vi "setRampTime.vi"(8 "error in (no error)":errorcluster, 10 "rampTime":dbl, 11 "RfRamp in":refnum<class "RfRamp.lvclass">) -> (0 "error out":errorcluster, 3 "RfRamp out":refnum<class "RfRamp.lvclass">)   [LabVIEW 2011, in "Tools.lvlib" / "Scripting.lvlib" / "RfRamp.lvclass"]
uses:
  RfRamp.lvclass
  RfRamp.lvclass/RfRamp.ctl
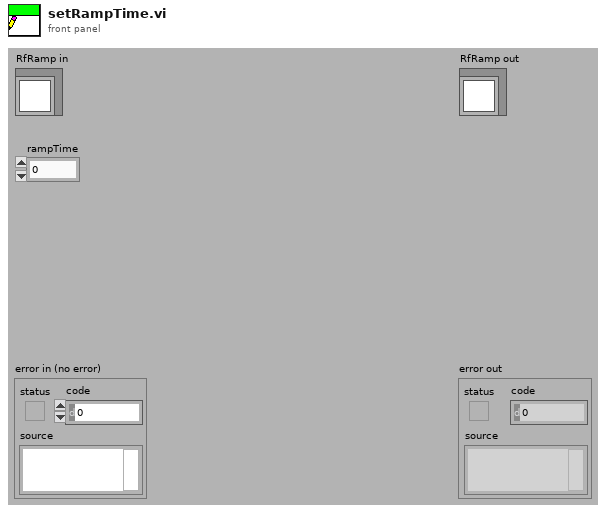
[diagram p1: front panel]
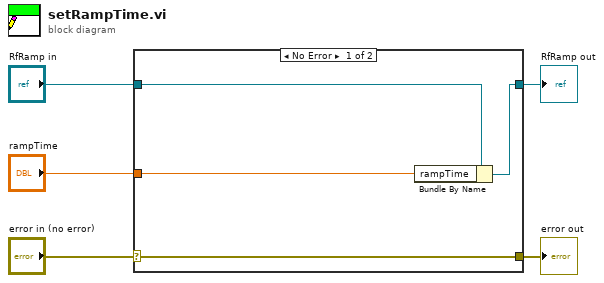
[diagram p0: block diagram]
diagram:
  n1 = case shown="No Error" "error in (no error)" {
    selector: "error in (no error)" -> [w9 w10]
    tunnel: [w9 w10] -> w4
    tunnel: [w7 w11] -> w2
    tunnel: "RfRamp in" -> [w8 w11]
    tunnel: "rampTime" -> [w6 _]
    frame No Error {
      n2 = Bundle By Name(cluster=w8, "rampTime"=w6) -> (w7:refnum<class "RfRamp.lvclass">)
    }
    frame Error {
    }
  }
  "error out" <- w4
  "RfRamp out" <- w2
